vi "split-json-4-ways.vi"(11 "json-string-in":string) -> (0 "sensor-json":string, 1 "serial-json":string, 2 "datalogging-json":string, 3 "filepath-json":string)   [LabVIEW 2024]
uses:
  <vilib>/regexp/Match Regular Expression.xnode
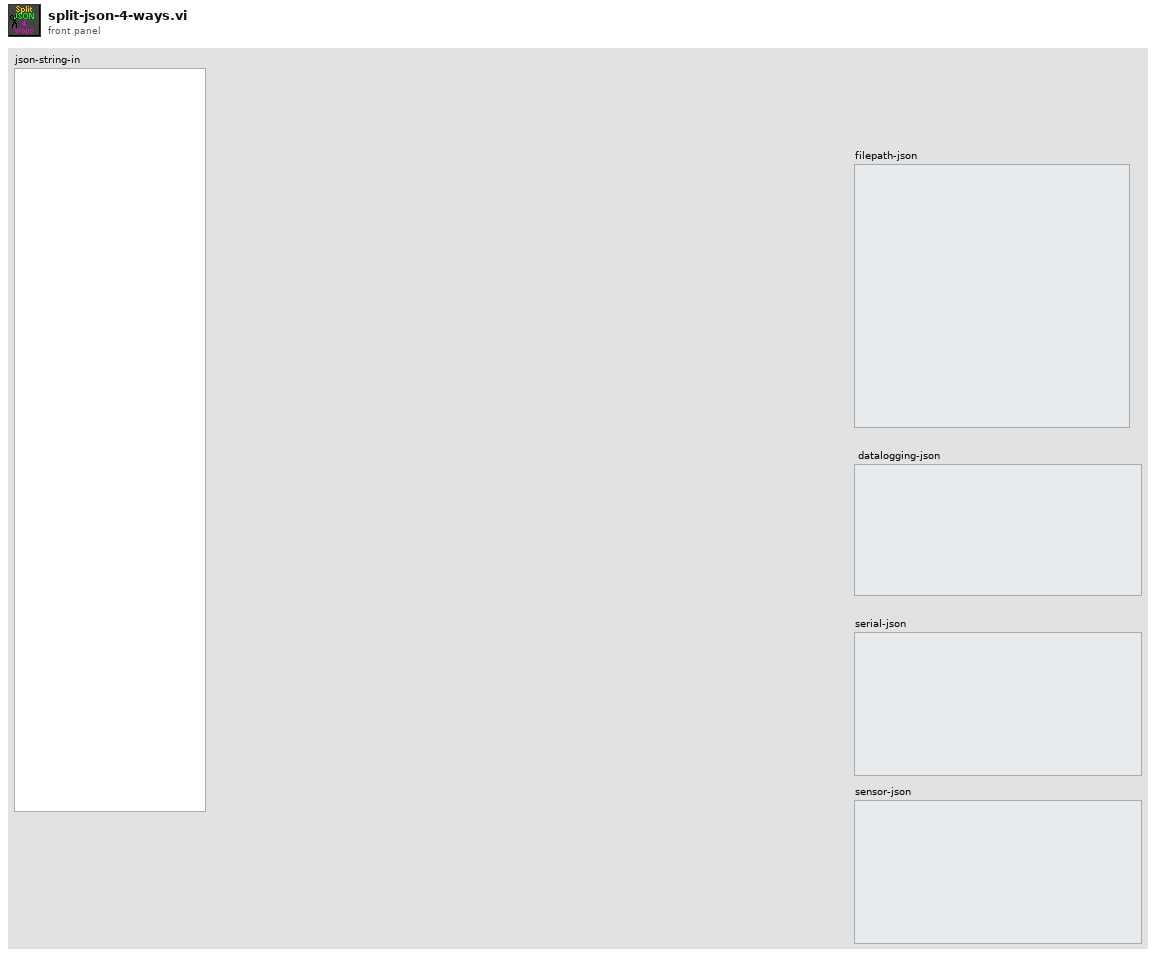
[diagram p1: front panel]
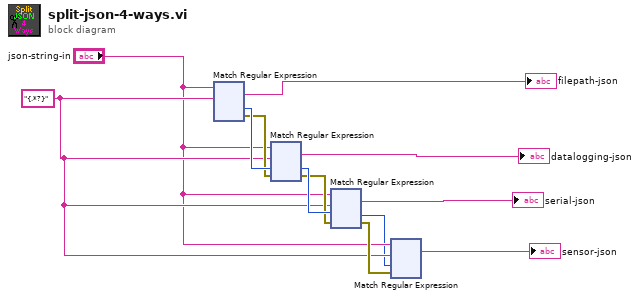
[diagram p0: block diagram]
diagram:
  w4 = "{.*?}" ("regular expression")
  n1 = xnode "Match Regular Expression"("input string"="json-string-in", "regular expression"=w4) -> ("whole match"=→"filepath-json":string, "offset past match"=w11:i32, "error out"=w8:errorcluster)  [unwired: 4 in, 2 out]
  n2 = xnode "Match Regular Expression"("input string"="json-string-in", "regular expression"=w4, "offset (0)"=w11, "error in"=w8) -> ("whole match"=→"datalogging-json":string, "offset past match"=w9:i32, "error out"=w7:errorcluster)  [unwired: 2 in, 2 out]
  n3 = xnode "Match Regular Expression"("input string"="json-string-in", "regular expression"=w4, "offset (0)"=w9, "error in"=w7) -> ("whole match"=→"serial-json":string, "offset past match"=w2:i32, "error out"=w5:errorcluster)  [unwired: 2 in, 2 out]
  n4 = xnode "Match Regular Expression"("input string"="json-string-in", "regular expression"=w4, "offset (0)"=w2, "error in"=w5) -> ("whole match"=→"sensor-json":string)  [unwired: 2 in, 4 out]
